vi "LowpassFilter.vi"(1 "Ts [ms]":dbl, 2 "Tf [s]":dbl, 3 "Y(n)":dbl) -> (0 "Y(n+1)":dbl)   [LabVIEW 2021]
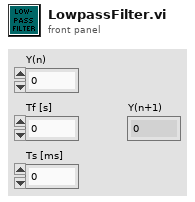
[diagram p1: front panel]
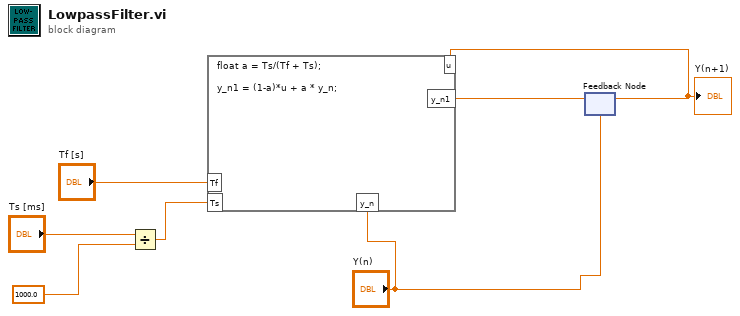
[diagram p0: block diagram]
diagram:
  n1 = Divide(x="Ts [ms]", y=1000.0) -> (x/y=w6:dbl)
  n2 = feedback #1("Y(n)") -> (w2:dbl)
  "Y(n+1)" <- w2
  n3 = formula code="float a = Ts/(Tf + Ts);\n \ny_n1 = (1-a)*u + a * y_n;"("y_n"="Y(n)", "Tf"="Tf [s]", "Ts"=w6, "u"=w2) -> ("y_n1"=w3:dbl)
  n4 = feedback-in #1(w3) -> ()
